vi "Create.vi"(8 "ErrorArray":errorcluster[](array[cluster]), 11 "TestBase.lvclass":refnum<class "TestBase.lvclass">) -> (0 "ErrorArray":errorcluster[](array[cluster]), 3 "TestBase.lvclass":refnum<class "TestBase.lvclass">)   [LabVIEW 2014, in "TestBase.lvclass"]
uses:
  TestBase.lvclass
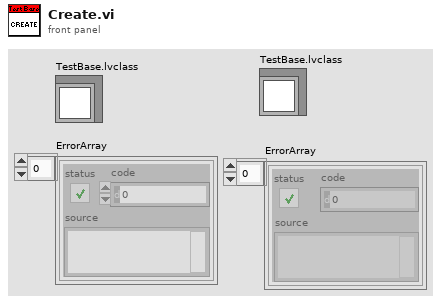
[diagram p1: front panel]
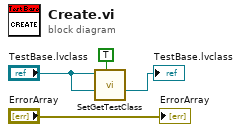
[diagram p0: block diagram]
diagram:
  n1 = call "SetGetTestClass.vi"("Set? (F)"=TRUE, "TestBase.lvclass"="TestBase.lvclass") -> ()  [unwired: 9 in, 1 out]
  "ErrorArray" <- "ErrorArray"
  "TestBase.lvclass" <- "TestBase.lvclass"
